vi "Launch TimerDRV.vi"(8 "error in (no error)":errorcluster, 11 "TimerDRV in":refnum<class "TimerDRV.lvclass">) -> (0 "error out":errorcluster, 3 "TimerDRV out":refnum<class "TimerDRV.lvclass">)   [LabVIEW 2019, in "TimingDRV Engine.lvlib" / "TimerDRV.lvclass"]
uses:
  TimerDRV.lvclass
  TimerDRV.lvclass/TimerDRV.ctl
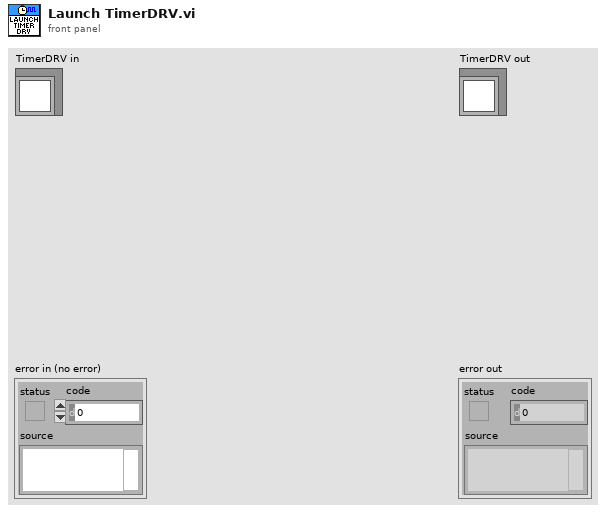
[diagram p1: front panel]
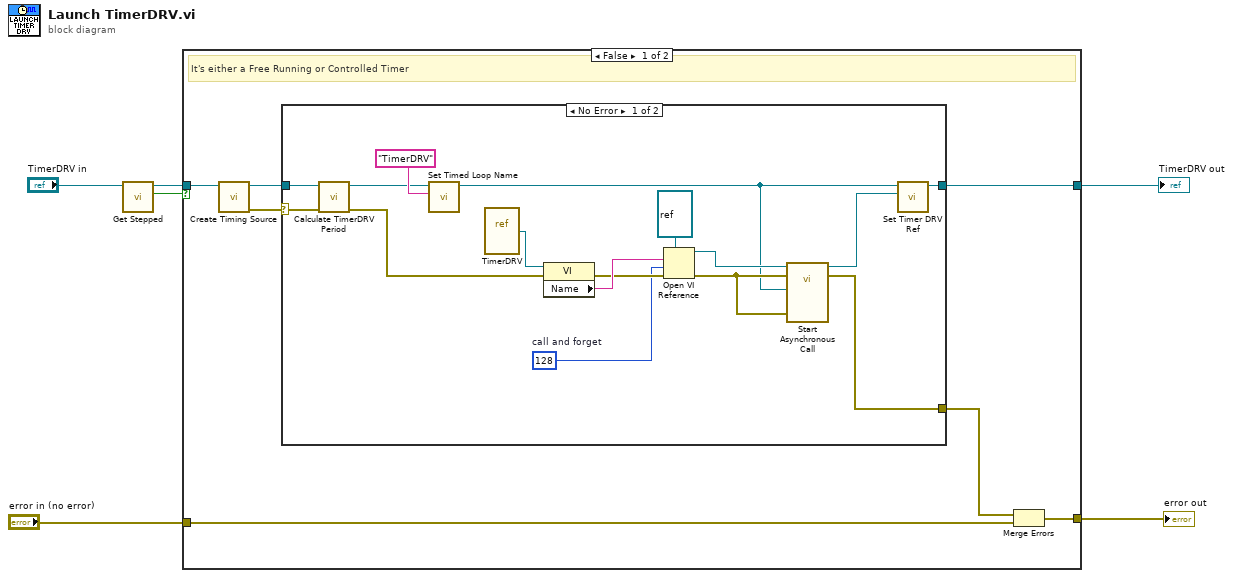
[diagram p0: block diagram]
diagram:
  n1 = call "Get Stepped.vi"("TimerDRV in"="TimerDRV in") -> ("Stepped"=w2:bool, "TimerDRV out"=w1:refnum<class "TimerDRV.lvclass">)  [unwired: 9 in]
  n2 = case shown="False" w2 {
    tunnel: [w13 w33] -> w6
    tunnel: "error in (no error)" -> [w9 w32]
    tunnel: [w8 w32] -> w4
    tunnel: w1 -> [w7 w33]
    frame False {
      # "It's either a Free Running or Controlled Timer"
      n3 = call "Create Timing Source.vi"("TimerDRV in"=w7) -> ("error out"=w11:errorcluster, "TimerDRV out"=w12:refnum<class "TimerDRV.lvclass">)  [unwired: 9 in]
      n4 = case shown="No Error" w11 {
        selector: w11 -> [w15 w30]
        tunnel: [w14 w30] -> w10
        tunnel: [w21 w31] -> w13
        tunnel: w12 -> [w18 w31]
        frame No Error {
          w24 = 128  # call and forget
          n5 = call "Calculate TimerDRV Period.vi"("error in (no error)"=w15, "TimerDRV in"=w18) -> ("error out"=w16:errorcluster, "TimerDRV out"=w17:refnum<class "TimerDRV.lvclass">)  [unwired: 8 in]
          n6 = call "Set Timed Loop Name.vi"("Timed Loop Name"="TimerDRV", "TimerDRV in"=w17) -> ("TimerDRV out"=w20:refnum<class "TimerDRV.lvclass">)  [unwired: 9 in]
          n7 = vi-ref "TimerDRV.vi"() -> (w27:refnum<vi>)
          n8 = property class="VI"(reference=w27, error in=w16) -> (error out=w25:errorcluster, "Name"=w26:string)  [unwired: 1 out]
          n9 = Open VI Reference(type specifier VI Refnum (for type only)=refnum<vi> refnum, vi path=w26, options=w24, error in (no error)=w25) -> (vi reference=w28:refnum<vi>, error out=w23:errorcluster)  [unwired: 2 in]
          n10 = call-by-ref "Start Asynchronous Call"(reference=w28, error in=w23, 8:"error in (no error)"=w23, "TimerDRV in"=w20) -> (reference out=w22:refnum<vi>, error out=w14:errorcluster)  [unwired: 8 in, 2 out]
          n11 = call "Set Timer DRV Ref.vi"("Timer DRV Ref"=w22, "TimerDRV in"=w20) -> ("TimerDRV out"=w21:refnum<class "TimerDRV.lvclass">)  [unwired: 9 in]
        }
        frame Error {
        }
      }
      n12 = Merge Errors(w10, w9) -> (w8:errorcluster)
    }
    frame True {
    }
  }
  "error out" <- w4
  "TimerDRV out" <- w6
